vi "KalmanFilter_Reset.vi"(11 "in KalmanFilter":T1) -> (3 "out KalmanFilter":T1)   [LabVIEW 2019, in "Trajectory_Library.lvlib"]
doc: "Resets xHat matrix to all zero\n\nInputs:\n - inKalmanFIlter -- filter data cluster\n\nOutpus:\n - outKalmanFilter -- filter data cluster"
uses:
  Trajectory_Library.lvlib
  TypeDef/KALMAN_FILTER.ctl
  <vilib>/Analysis/Matrix/Datatypes/RealMatrix.ctl
  TypeDef/LINEAR_SYSTEM.ctl
  <vilib>/Analysis/Matrix/NI_Matrix.lvlib
panel:
  # "Steady State Gain  \n<States,Outputs>"
  # "State Estimate <Statess,1>"
  # "<States,States>"
  # "<States,Inputs>"
  # "<Outputs,States>"
  # "<Outputs,Inputs>"
  # "Steady State Gain  \n<States,Outputs>"
  # "State Estimate <Statess,1>"
  # "<States,States>"
  # "<States,Inputs>"
  # "<Outputs,States>"
  # "<Outputs,Inputs>"
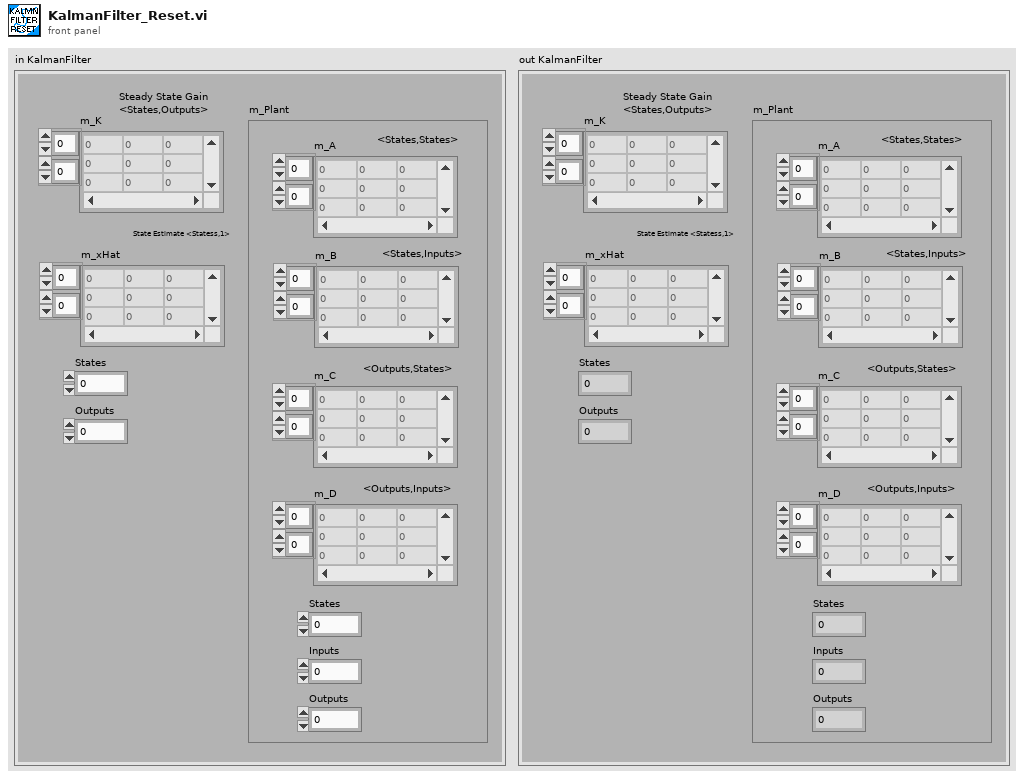
[diagram p1: front panel]
types:
  T1 = typedef "Trajectory_Library.lvlib/KALMAN_FILTER.ctl" = cluster{"m_K":T2, "m_xHat":T2, "States":i32, "Outputs":i32, "m_Plant":T3}
  T2 = typedef "NI_Matrix.lvlib/RealMatrix.ctl" = dbl[][]
  T3 = typedef "Trajectory_Library.lvlib/LINEAR_SYSTEM.ctl" = cluster{"m_A":T2, "m_B":T2, "m_C":T2, "m_D":T2, "States":i32, "Inputs":i32, "Outputs":i32}
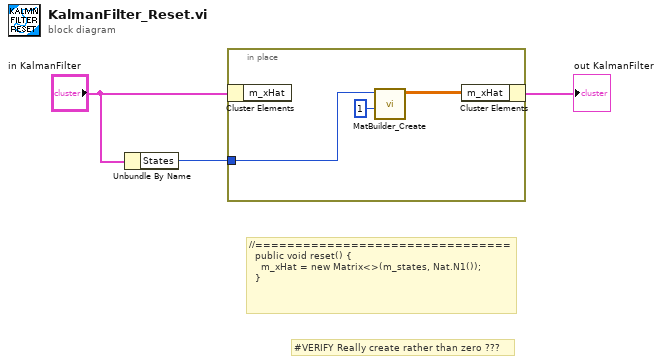
[diagram p0: block diagram]
diagram:
  # "#VERIFY Really create rather than zero ???"
  # "//================================\n  public void reset() {\n    m_xHat = new Matrix<>(m_states, Nat.N1());\n  }"
  n1 = Unbundle By Name("in KalmanFilter") -> ("States"=w1:i32)
  n2 = in-place {
    in-place-border: w1 -> [w6]
    n3 = in-place-cluster #1("in KalmanFilter") -> ()  [unwired: 1 out]
    n4 = call "MatBuilder_Create.vi"("Columns"=1, "Rows"=w6) -> ("output matrix"=w4:T2)  [unwired: 9 in]
    n5 = in-place-cluster #1("m_xHat"=w4) -> (→"out KalmanFilter":T1)
  }
